vi "enable and disable.vi"() -> ()   [LabVIEW 2020, in "UI Controls Manager.lvlib"]
uses:
  UI Controls Manager.lvlib
  uiControlsMgr.lvclass
panel:
  in  "Button":bool
  out "Waveform Chart":dbl(graph)
  in  "Boolean":bool
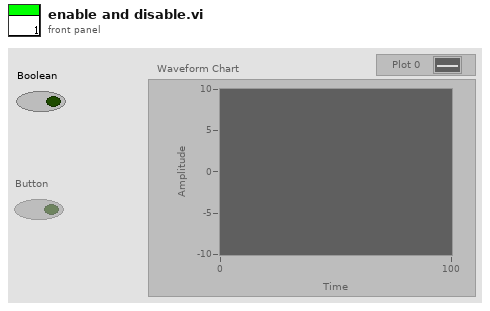
[diagram p1: front panel]
types:
  T1 = cluster{"label":string, "State":enum8{"Enabled", "Disabled", "Disabled and Grayed Out"}}[]
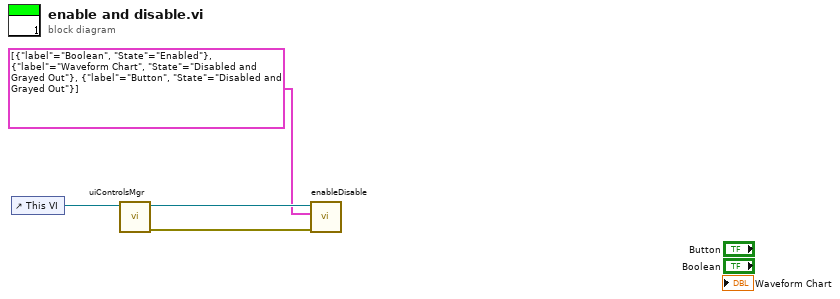
[diagram p0: block diagram]
diagram:
  n1 = control-ref of="This VI"() -> (w4:refnum<vi>)
  n2 = call "uiControlsMgr.vi"("VI reference"=w4) -> ("error out"=w2:errorcluster, "uiControlsMgr out"=w3:refnum<class "uiControlsMgr.lvclass">)  [unwired: 9 in]
  n3 = call "enableDisable.vi"("error in (no error)"=w2, "Controls - Status"=T1 [{"label"="Boolean", "State"=enum."Enabled"}, {"label"="Waveform Chart", "State"=enum."Disabled and Grayed Out"}, {"label"="Button", "State"=enum."Disabled and Grayed Out"}], "uiControlsMgr in"=w3) -> ()  [unwired: 7 in, 2 out]
